vi "Drive Saftey.vi"(11 "Operation States":T2) -> (3 "Operation States":T2)   [LabVIEW 2014]
uses:
  <vilib>/Rock Robotics/WPI/Solenoid/WPI_SolenoidValue.ctl
  Robot Global Data.vi
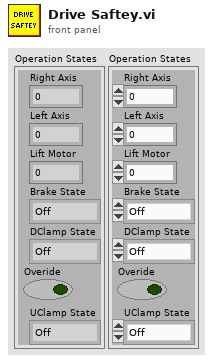
[diagram p1: front panel]
types:
  T1 = typedef "WPI_SolenoidValue.ctl" = enum16{"Off", "On", "Forward", "Reverse"}
  T2 = cluster{"Right Axis":dbl, "Left Axis":dbl, "Lift Motor":dbl, "Brake State":T1, "DClamp State":T1, "Overide":bool, "UClamp State":T1}
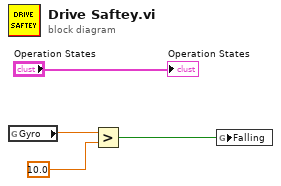
[diagram p0: block diagram]
diagram:
  n1 = global read "Robot Global Data.vi" "Gyro"() -> (w4:dbl)
  n2 = Greater?(x=w4, y=10.0) -> (0:w3:bool)
  n3 = global write "Robot Global Data.vi" "Falling"(w3) -> ()
  "Operation States" <- "Operation States"
